vi "Obtain Plugin Interface.vi"(8 "error in (no error)":errorcluster, 9 "timeout in ms (0)":i32 format="%d ms", 11 "Plugin Interface Pool in":refnum<class "Plugin Interface Pool.lvclass">) -> (0 "error out":errorcluster, 1 "timed out?":bool, 2 "Plugin Interface":refnum<class "Plugin Interface.lvclass">, 3 "Plugin Interface Pool out":refnum<class "Plugin Interface Pool.lvclass">)   [LabVIEW 2017, in "DSF Core.lvlib" / "Plugin Interface Pool.lvclass"]
uses:
  Plugin Interface Pool.lvclass
  C:/Git/DSF/Core/Classes/Pool/Pool.lvclass
  Interface/Plugin/Plugin Interface.lvclass
  Plugin Interface Pool.lvclass/Plugin Interface Pool.ctl
  Pool.lvclass
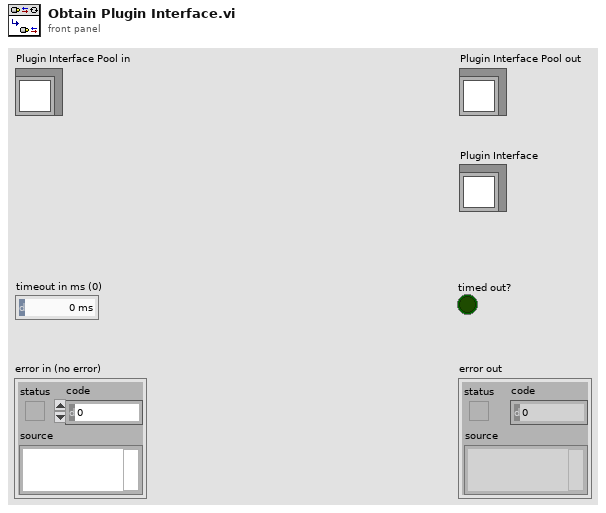
[diagram p1: front panel]
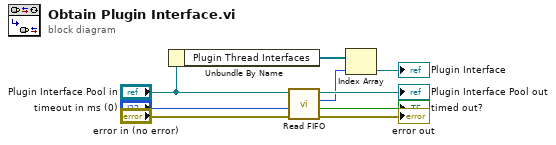
[diagram p0: block diagram]
diagram:
  n1 = Unbundle By Name("Plugin Interface Pool in") -> ("Plugin Thread Interfaces"=w4:refnum<class "Plugin Interface.lvclass">[])
  n2 = call "Read FIFO.vi"("error in (no error)"="error in (no error)", "timeout in ms (0)"="timeout in ms (0)", "Pool in"="Plugin Interface Pool in") -> ("error out"=→"error out":errorcluster, "timed out?"=→"timed out?":bool, "element"=w3:i32, "Pool out"=→"Plugin Interface Pool out":refnum<class "Plugin Interface Pool.lvclass">)  [unwired: 5 in]
  n3 = Index Array(array=w4, index=w3) -> (element=→"Plugin Interface":refnum<class "Plugin Interface.lvclass">)
